vi "LabVIEW-ESP32 TCP Example.vi"() -> ()   [LabVIEW 2021]
doc: "Demonstrates how to open a connection to an TCP server, read the data being sent, and display the data on a chart. This VI is designed to stop if the TCP connection is terminated."
panel:
  in  "stop":bool
  in  "Negative Button":bool
  in  "Positive Button":bool
  out "Waveform Graph":waveform(i16)[](graph)
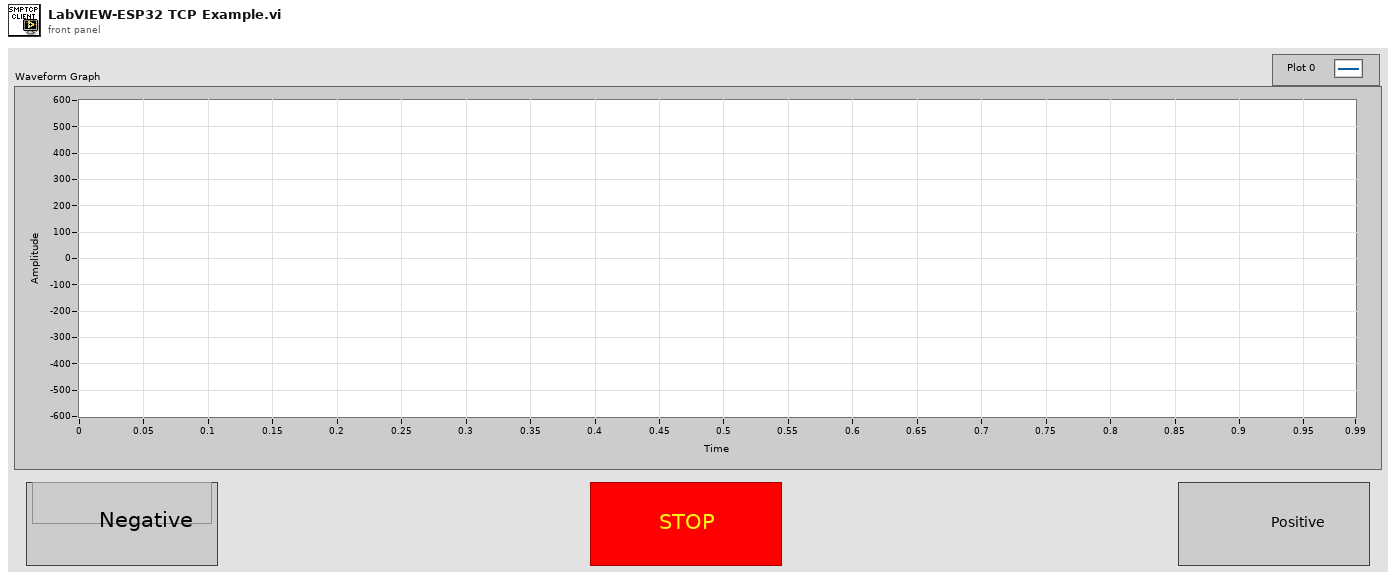
[diagram p1: front panel]
types:
  T1 = enum16{"Standard", "Buffered", "CRLF", "Immediate"}
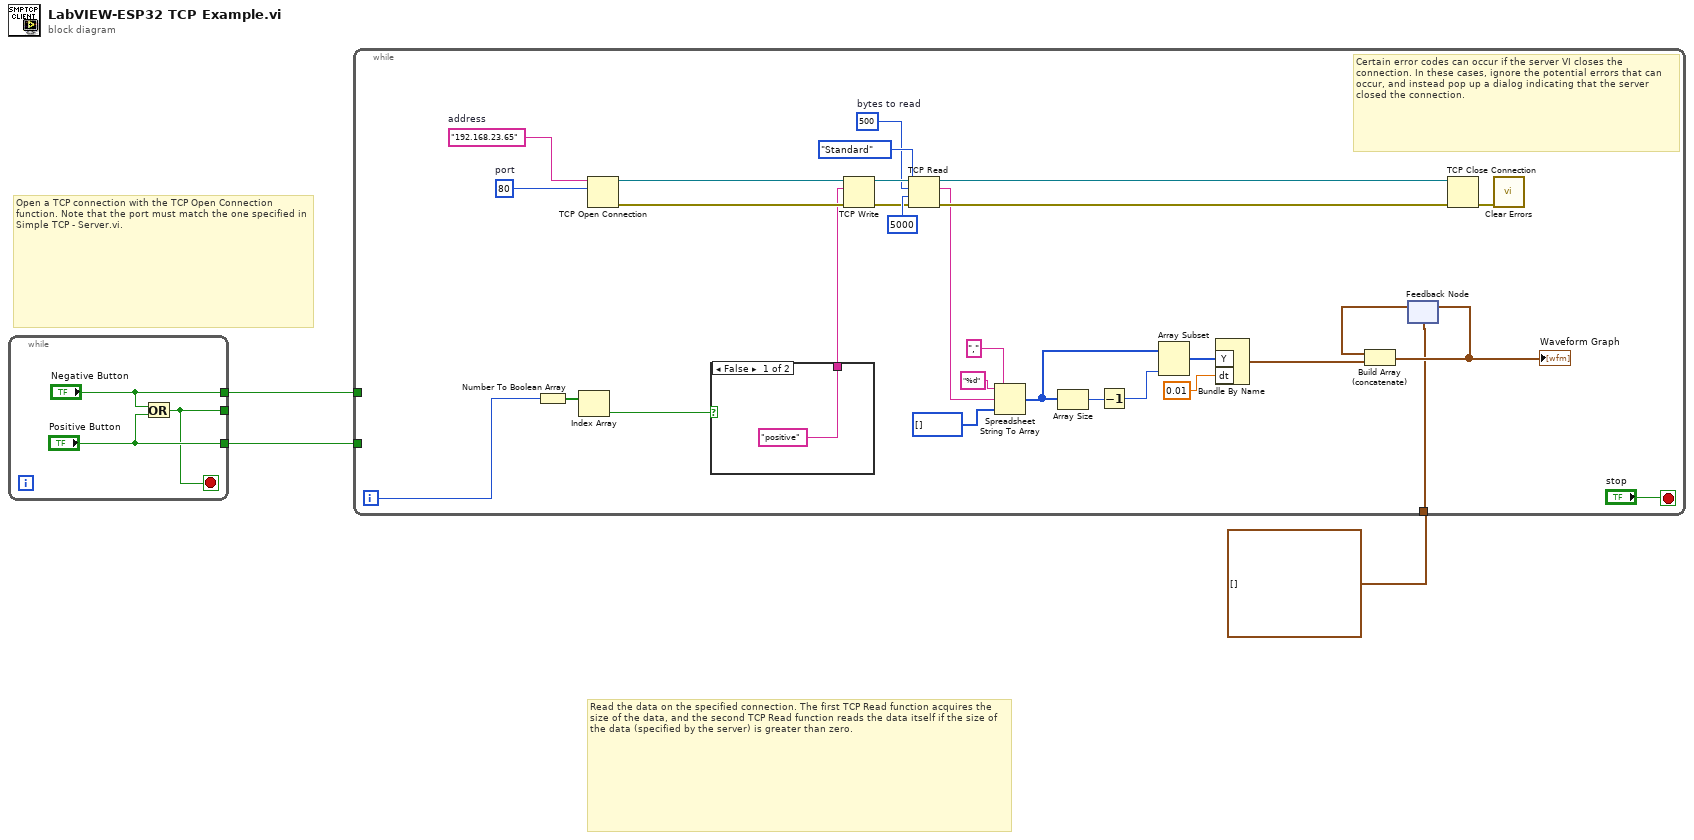
[diagram p0: block diagram]
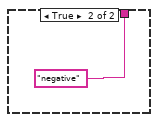
[diagram p2: hidden frame]
diagram:
  # "Read the data on the specified connection. The first TCP Read function acquires the size of the data, and the second TCP Read function reads the data itself if the size of the data (specified by the server) is greater than zero."
  # "Open a TCP connection with the TCP Open Connection function. Note that the port must match the one specified in Simple TCP - Server.vi."
  n1 = while {
    tunnel: [w4] -> _
    tunnel: ["Negative Button"] -> w3
    tunnel: ["Positive Button"] -> w2
    stop <- w4 stop-if-true
    n2 = Or(x="Negative Button", y="Positive Button") -> (x .or. y?=w4:bool)
  }
  n3 = while {
    tunnel: w3 -> [_]
    tunnel: w2 -> [_]
    tunnel: waveform(i16)[] [] ("Waveform Graph") -> [w7]
    i -> [w10]
    stop <- "stop" stop-if-true
    w24 = 500  # bytes to read
    w33 = u16 80  # port
    w34 = "192.168.23.65"  # address
    # "Certain error codes can occur if the server VI closes the connection. In these cases, ignore the potential errors that can occur, and instead pop up a dialog indicating that the server closed the connection."
    n4 = Number To Boolean Array(number=w10) -> (Boolean array=w9:bool[])
    n5 = Index Array(array=w9) -> (element=w8:bool)  [unwired: 1 in]
    n6 = TCP Open Connection(address=w34, remote port or service name=w33) -> (connection ID=w36:refnum<k5>, error out=w35:errorcluster)  [unwired: 3 in]
    n7 = case shown="False" w8 {
      tunnel: ["positive" ("data in") "negative" ("data in")] -> w26
      frame False {
      }
      frame True {
      }
    }
    n8 = TCP Write(connection ID=w36, data in=w26, error in (no error)=w35) -> (connection ID out=w27:refnum<k5>, error out=w28:errorcluster)  [unwired: 1 in, 1 out]
    n9 = TCP Read(connection ID=w27, bytes to read=w24, error in (no error)=w28, 7:T1."Standard" ("mode (standard)"), 9:5000 ("timeout ms (25000)")) -> (connection ID out=w32:refnum<k5>, data out=w23:string, error out=w31:errorcluster)
    n10 = Spreadsheet String To Array(delimiter (Tab)=",", format string="%d", spreadsheet string=w23, array type (2D Dbl)=i16[] []) -> (array=w18:i16[])
    n11 = Array Size(array=w18) -> (size(s)=w19:i32)
    n12 = Decrement(x=w19) -> (x-1=w17:i32)
    n13 = Array Subset(array=w18, length=w17) -> (w16:i16[])  [unwired: 1 in]
    n14 = Bundle By Name("Y"=w16, "dt"=0.01) -> (w14:waveform(i16))  [unwired: 1 in]
    n15 = feedback #1(w7) -> (w13:waveform(i16)[])
    n16 = Build Array (concatenate)(w13, w14) -> (w12:waveform(i16)[])
    "Waveform Graph" <- w12
    n17 = feedback-in #1(w12) -> ()
    n18 = TCP Close Connection(connection ID=w32, error in (no error)=w31) -> (error out=w30:errorcluster)  [unwired: 1 in, 1 out]
    n19 = call <vilib>:"Clear Errors.vi"("error in (no error)"=w30) -> ()  [unwired: 5 in, 2 out]
  }
